vi "DriveBase.vi"(9 "Elevator State":string="Hatch_Rocket_1") -> ()   [LabVIEW 2018]
uses:
  RobotStates.vi
  Inputs_DriverStation.vi
  SensorReadings.vi
panel:
  in  "Forward Acceleration (p/s)":dbl=10.0
  in  "Time Above Speed (ms)":u32=100
  in  "Stabilization Height (in)":dbl=36.0
  in  "Switch to Low Gear (ft/s)":dbl=0.5
  in  "Switch to High Gear (ft/s)":dbl=6.0
  in  "Elevator Danger Height (in)":dbl=52.0
  in  "Backward Acceleration (p/s)":dbl=1.0
  in  "Climb-Drive Bias":dbl=-0.4
  in  "Turning Deadband":dbl=0.2
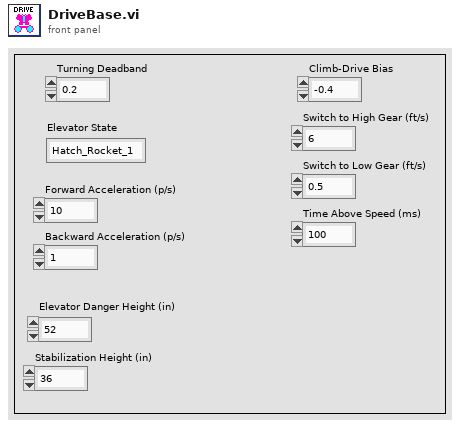
[diagram p1: front panel]
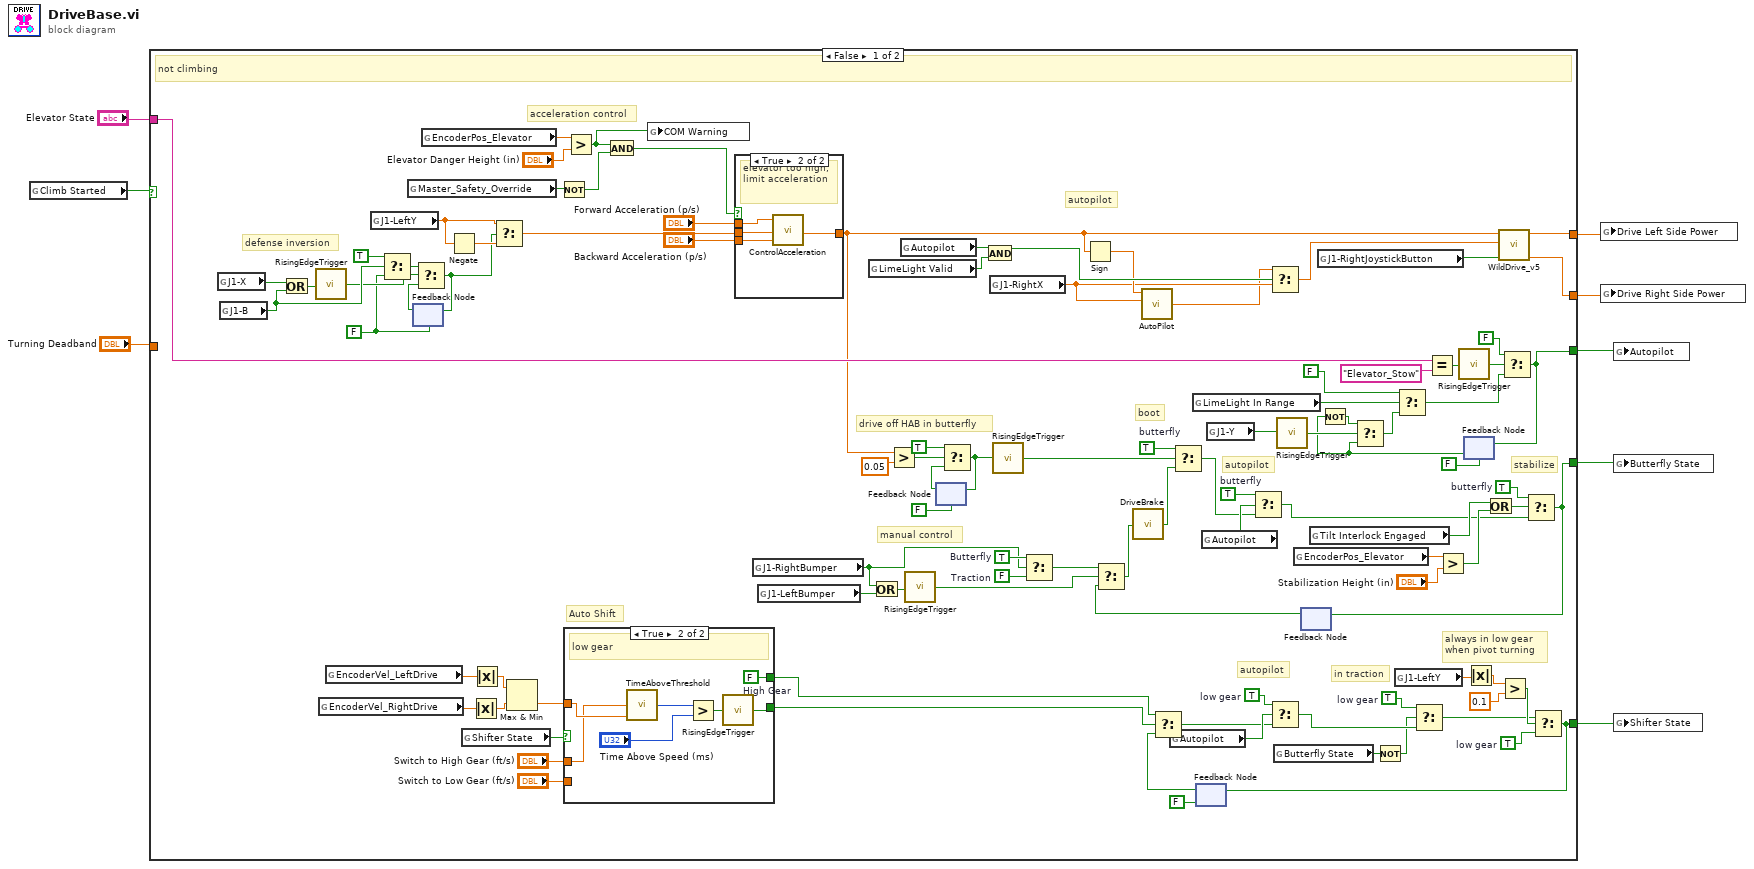
[diagram p0: block diagram]
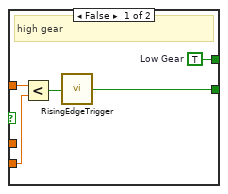
[diagram p2: hidden frame]
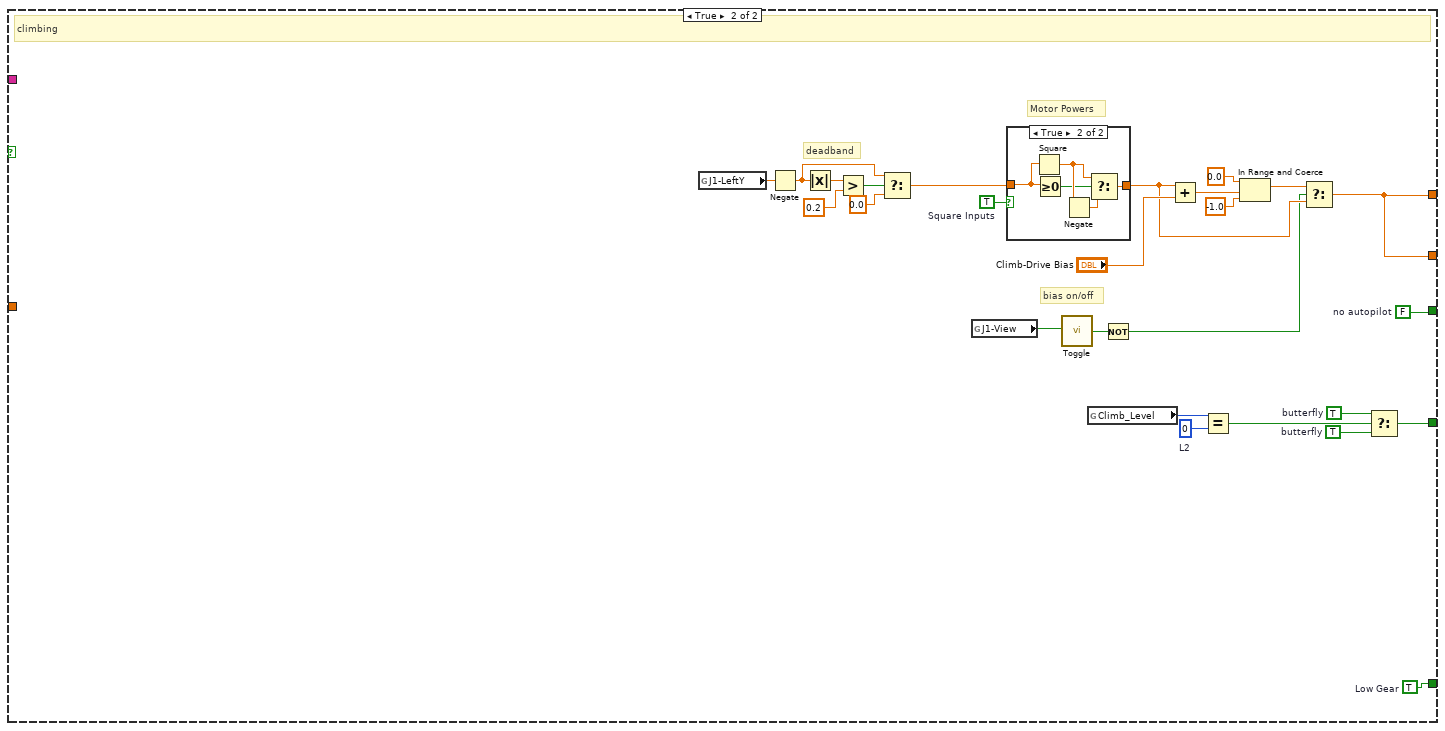
[diagram p4: hidden frame]
diagram:
  n1 = global read "RobotStates.vi" "Climb Started"() -> (w5:bool)
  n2 = case shown="False" w5 {
    tunnel: [w73 w133] -> w8
    tunnel: [w63 w152] -> w7
    tunnel: "Turning Deadband" -> [_ _]
    tunnel: [w15 w135] -> w1
    tunnel: [w14 w135] -> w2
    tunnel: [w42 w134] -> w4
    tunnel: "Elevator State" -> [w41 _]
    frame False {
      w19 = FALSE
      w31 = TRUE  # low gear
      w53 = TRUE  # butterfly
      w56 = TRUE  # low gear
      w62 = TRUE  # low gear
      w74 = FALSE  # Traction
      w75 = TRUE  # Butterfly
      w81 = TRUE  # butterfly
      w88 = TRUE  # butterfly
      # "defense inversion"
      # "in traction"
      # "acceleration control"
      # "always in low gear\nwhen pivot turning"
      # "autopilot"
      # "stabilize"
      # "autopilot"
      # "boot"
      # "manual control"
      # "autopilot"
      # "drive off HAB in butterfly"
      # "Auto Shift"
      # "not climbing"
      n3 = global read "Inputs_DriverStation.vi" "J1-X"() -> (w64:bool)
      n4 = global read "Inputs_DriverStation.vi" "J1-B"() -> (w24:bool)
      n5 = Or(x=w64, y=w24) -> (x .or. y?=w109:bool)
      n6 = call "RisingEdgeTrigger.vi"("Raw Signal"=w109) -> ("Trigger"=w21:bool)
      n7 = global read "SensorReadings.vi" "EncoderVel_RightDrive"() -> (w96:dbl)
      n8 = global read "SensorReadings.vi" "EncoderVel_LeftDrive"() -> (w97:dbl)
      n9 = global read "Inputs_DriverStation.vi" "J1-LeftY"() -> (w12:dbl)
      n10 = Select(t=TRUE, s=w24, f=w19) -> (s? t:f=w22:bool)
      n11 = global read "Inputs_DriverStation.vi" "Master_Safety_Override"() -> (w100:bool)
      n12 = feedback #1(w19) -> (w20:bool)
      n13 = Select(t=w22, s=w21, f=w20) -> (s? t:f=w10:bool)
      n14 = feedback-in #1(w10) -> ()
      n15 = global read "SensorReadings.vi" "EncoderPos_Elevator"() -> (w103:dbl)
      n16 = Negate(x=w12) -> (-x=w13:dbl)
      n17 = global read "RobotStates.vi" "Shifter State"() -> (w95:bool)
      n18 = Absolute Value(x=w96) -> (abs(x)=w90:dbl)
      n19 = Absolute Value(x=w97) -> (abs(x)=w91:dbl)
      n20 = Select(t=w12, s=w10, f=w13) -> (s? t:f=w18:dbl)
      n21 = Max & Min(x=w91, y=w90) -> (min(x,y)=w69:dbl)  [unwired: 1 out]
      n22 = Not(x=w100) -> (.not. x?=w99:bool)
      n23 = case shown="True" w95 {
        tunnel: w69 -> [w114 w116]
        tunnel: "Switch to High Gear (ft/s)" -> [_ w115]
        tunnel: "Switch to Low Gear (ft/s)" -> [w113 _]
        tunnel: [w110 w120] -> w89
        tunnel: [w112 w121] -> w92
        frame False {
          w112 = TRUE  # Low Gear
          # "high gear"
          n24 = Less?(x=w114, y=w113) -> (x < y?=w111:bool)
          n25 = call "RisingEdgeTrigger.vi"("Raw Signal"=w111) -> ("Trigger"=w110:bool)
        }
        frame True {
          w121 = FALSE  # High Gear
          # "low gear"
          n26 = call "TimeAboveThreshold.vi"("Current Value"=w116, "Threshold"=w115) -> ("Time Above"=w119:u32)  [unwired: 3 in]
          n27 = Greater?(x=w119, y="Time Above Speed (ms)") -> (0:w117:bool)
          n28 = call "RisingEdgeTrigger.vi"("Raw Signal"=w117) -> ("Trigger"=w120:bool)
        }
      }
      n29 = Greater?(x=w103, y="Elevator Danger Height (in)") -> (0:w98:bool)
      n30 = And(x=w98, y=w99) -> (x .and. y?=w101:bool)
      n31 = global write "RobotStates.vi" "COM Warning"(w98) -> ()
      n32 = case shown="True" w101 {
        tunnel: w18 -> [w122 w126]
        tunnel: [w122 w125] -> w17
        tunnel: "Backward Acceleration (p/s)" -> [_ w124]
        tunnel: "Forward Acceleration (p/s)" -> [_ w123]
        frame False {
          # "elevator down"
        }
        frame True {
          # "elevator too high, limit acceleration"
          n33 = call "ControlAcceleration.vi"("Backward Acceleration (p/s)"=w124, "Raw"=w126, "Forward Acceleration (p/s)"=w123) -> ("Controlled"=w125:dbl)
        }
      }
      n34 = global read "Inputs_DriverStation.vi" "J1-RightBumper"() -> (w71:bool)
      n35 = global read "Inputs_DriverStation.vi" "J1-LeftBumper"() -> (w72:bool)
      n36 = global read "SensorReadings.vi" "LimeLight Valid"() -> (w105:bool)
      n37 = Or(x=w71, y=w72) -> (x .or. y?=w79:bool)
      n38 = Greater?(x=w17, y=0.05) -> (0:w83:bool)
      n39 = global read "RobotStates.vi" "Autopilot"() -> (w107:bool)
      n40 = call "RisingEdgeTrigger.vi"("Raw Signal"=w79) -> ("Trigger"=w76:bool)
      n41 = feedback #2(FALSE) -> (w86:bool)
      n42 = Select(t=TRUE, s=w83, f=w86) -> (s? t:f=w85:bool)
      n43 = feedback-in #2(w85) -> ()
      n44 = And(x=w107, y=w105) -> (x .and. y?=w106:bool)
      n45 = global read "Inputs_DriverStation.vi" "J1-RightX"() -> (w26:dbl)
      n46 = call "RisingEdgeTrigger.vi"("Raw Signal"=w85) -> ("Trigger"=w70:bool)
      n47 = Select(t=w75, s=w71, f=w74) -> (s? t:f=w77:bool)
      n48 = Sign(1:w17) -> (0:w50:dbl)
      n49 = call "AutoPilot.vi"("Human Contribution"=w26, "Drive Direction"=w50) -> ("End Contribution"=w11:dbl)  [unwired: 2 in]
      n50 = global read "RobotStates.vi" "Autopilot"() -> (w57:bool)
      n51 = global read "SensorReadings.vi" "LimeLight In Range"() -> (w34:bool)
      n52 = feedback #3(FALSE ("Low Gear")) -> (w25:bool)
      n53 = Select(t=w92, s=w89, f=w25) -> (s? t:f=w55:bool)
      n54 = global read "RobotStates.vi" "Autopilot"() -> (w54:bool)
      n55 = global read "Inputs_DriverStation.vi" "J1-Y"() -> (w43:bool)
      n56 = Select(t=w11, s=w106, f=w26) -> (s? t:f=w16:dbl)
      n57 = Select(t=w56, s=w57, f=w55) -> (s? t:f=w30:bool)
      n58 = global read "RobotStates.vi" "Butterfly State"() -> (w28:bool)
      n59 = call "RisingEdgeTrigger.vi"("Raw Signal"=w43) -> ("Trigger"=w46:bool)
      n60 = global read "SensorReadings.vi" "EncoderPos_Elevator"() -> (w68:dbl)
      n61 = feedback #4() -> (w78:bool)  [unwired: 1 in]
      n62 = Select(t=w77, s=w76, f=w78) -> (s? t:f=w36:bool)
      n63 = call "DriveBrake.vi"("Butterfly State In"=w36) -> ("Butterfly State Out"=w37:bool)
      n64 = Select(t=w88, s=w70, f=w37) -> (s? t:f=w52:bool)
      n65 = Select(t=w53, s=w54, f=w52) -> (s? t:f=w51:bool)
      n66 = global read "RobotStates.vi" "Tilt Interlock Engaged"() -> (w65:bool)
      n67 = global read "Inputs_DriverStation.vi" "J1-RightJoystickButton"() -> (w9:bool)
      n68 = Not(x=w28) -> (.not. x?=w27:bool)
      n69 = global read "Inputs_DriverStation.vi" "J1-LeftY"() -> (w61:dbl)
      n70 = Select(t=w31, s=w27, f=w30) -> (s? t:f=w29:bool)
      n71 = Equal?(x=w41, y="Elevator_Stow") -> (x = y?=w39:bool)
      n72 = Greater?(x=w68, y="Stabilization Height (in)") -> (0:w66:bool)
      n73 = call "RisingEdgeTrigger.vi"("Raw Signal"=w39) -> ("Trigger"=w38:bool)
      n74 = feedback #5(FALSE) -> (w44:bool)
      n75 = Not(x=w44) -> (.not. x?=w45:bool)
      n76 = Select(t=w45, s=w46, f=w44) -> (s? t:f=w33:bool)
      n77 = Select(t=FALSE, s=w34, f=w33) -> (s? t:f=w32:bool)
      n78 = Absolute Value(x=w61) -> (abs(x)=w60:dbl)
      n79 = Or(x=w65, y=w66) -> (x .or. y?=w80:bool)
      n80 = call "WildDrive_v5.vi"("Super Turn"=w9, "Turn Joystick"=w16, "Speed Joystick"=w17) -> ("Right Side Power"=w14:dbl, "Left Side Power"=w15:dbl)  [unwired: 7 in]
      n81 = Greater?(x=w60, y=0.1) -> (0:w59:bool)
      n82 = Select(t=FALSE, s=w38, f=w32) -> (s? t:f=w42:bool)
      n83 = feedback-in #5(w42) -> ()
      n84 = Select(t=w81, s=w80, f=w51) -> (s? t:f=w73:bool)
      n85 = feedback-in #4(w73) -> ()
      n86 = Select(t=w29, s=w59, f=w62) -> (s? t:f=w63:bool)
      n87 = feedback-in #3(w63) -> ()
    }
    frame True {
      w129 = u8 0  # L2
      w131 = TRUE  # butterfly
      w134 = FALSE  # no autopilot
      w146 = TRUE  # Square Inputs
      w152 = TRUE  # Low Gear
      w132 = TRUE  # butterfly
      # "deadband"
      # "bias on/off"
      # "Motor Powers"
      # "climbing"
      n88 = global read "Inputs_DriverStation.vi" "J1-LeftY"() -> (w149:dbl)
      n89 = Negate(x=w149) -> (-x=w150:dbl)
      n90 = Absolute Value(x=w150) -> (abs(x)=w147:dbl)
      n91 = Greater?(x=w147, y=0.2) -> (0:w148:bool)
      n92 = Select(t=w150, s=w148, f=0.0) -> (s? t:f=w151:dbl)
      n93 = global read "Inputs_DriverStation.vi" "J1-View"() -> (w140:bool)
      n94 = case shown="True" w146 {
        tunnel: [w153 w158] -> w137
        tunnel: w151 -> [w153 w157]
        frame False {
        }
        frame True {
          n95 = Square(x=w157) -> (x^2=w155:dbl)
          n96 = Greater Or Equal To 0?(x=w157) -> (x >= 0?=w154:bool)
          n97 = Negate(x=w155) -> (-x=w156:dbl)
          n98 = Select(t=w155, s=w154, f=w156) -> (s? t:f=w158:dbl)
        }
      }
      n99 = call "Toggle.vi"("Trigger"=w140) -> ("New Mode"=w139:bool)
      n100 = global read "Inputs_DriverStation.vi" "Climb_Level"() -> (w130:u8)
      n101 = Not(x=w139) -> (.not. x?=w136:bool)
      n102 = Add(x=w137, y="Climb-Drive Bias") -> (x+y=w144:dbl)
      n103 = Equal?(x=w130, y=w129) -> (x = y?=w128:bool)
      n104 = In Range and Coerce(upper limit=0.0, x=w144, lower limit=-1.0) -> (coerced(x)=w138:dbl)  [unwired: 1 out]
      n105 = Select(t=w138, s=w136, f=w137) -> (s? t:f=w135:dbl)
      n106 = Select(t=w131, s=w128, f=w132) -> (s? t:f=w133:bool)
    }
  }
  n107 = global write "RobotStates.vi" "Drive Left Side Power"(w1) -> ()
  n108 = global write "RobotStates.vi" "Drive Right Side Power"(w2) -> ()
  n109 = global write "RobotStates.vi" "Autopilot"(w4) -> ()
  n110 = global write "RobotStates.vi" "Butterfly State"(w8) -> ()
  n111 = global write "RobotStates.vi" "Shifter State"(w7) -> ()
